vi "Add Battery Switch card.vi"(8 "error in (no error)":errorcluster, 11 "Node Ptr":u64 format="%.0x") -> (0 "error out":errorcluster)   [LabVIEW 2014, in "SLSC configuration System Explorer.lvlib"]
uses:
  SLSC configuration System Explorer.lvlib
  Shared/Constants.vi
  Shared/SLSC configuration Shared.lvlib
panel:
  in  "Tag":string
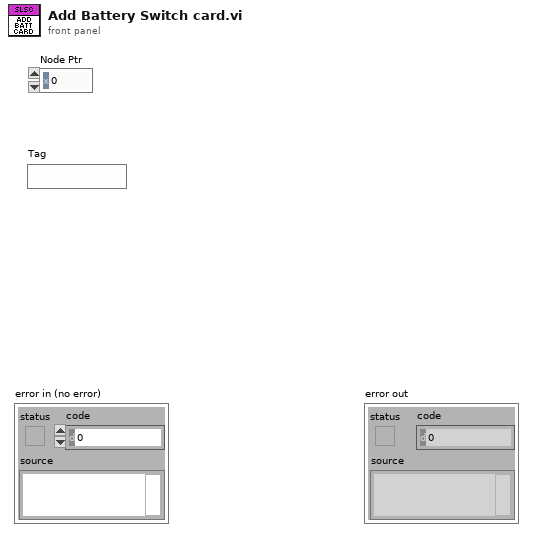
[diagram p1: front panel]
types:
  T1 = typedef "SLSC configuration Shared.lvlib/Card Position.ctl" = cluster{"Rack #":u8, "Slot #":T2}
  T2 = typedef "SLSC configuration Shared.lvlib/Slot #.ctl" = u8
  T3 = typedef "Custom Device API.lvlib/Custom Device Item Ref.ctl" = u64
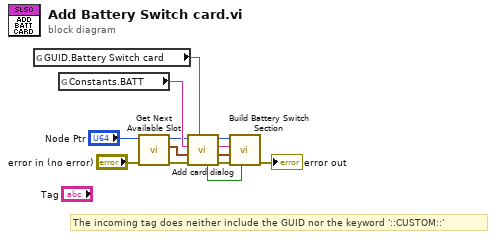
[diagram p0: block diagram]
diagram:
  # "The incoming tag does neither include the GUID nor the keyword '::CUSTOM::'"
  n1 = global read "Constants.vi" "GUID.Battery Switch card"() -> (w1:string)
  n2 = global read "Constants.vi" "Constants.BATT"() -> (w13:string)
  n3 = call "Get Next Available Slot.vi"("error in (no error)"="error in (no error)", "Device Ref in"="Node Ptr") -> ("error out"=w5:errorcluster, "Next Open Slot"=w7:T1, "Device Ref out"=w3:T3)  [unwired: 7 in]
  n4 = call "Add card dialog.vi"("Card GUID"=w1, "error in (no error)"=w5, "Card Position"=w7, "Card Type in"=w13, "Node Ptr"=w3) -> ("error out"=w12:errorcluster, "Card Position out"=w10:T1, "Name out"=w8:string, "Node Ptr out"=w11:u64, "Cancelled?"=w2:bool)  [unwired: 2 in]
  n5 = call "Build Battery Switch Section.vi"("Cancelled?"=w2, "error in (no error)"=w12, "Card Position in"=w10, "Name in"=w8, "Node Ptr in"=w11) -> ("error out"=→"error out":errorcluster)  [unwired: 6 in]
